vi "CALC_LIM_SEGM_AMPL_STOP.vi"(0 "VISA IN":refnum<visa-resource-name>, 1 "Segment number":i32, 2 "Stop number":i32, 5 "error in":errorcluster, 7 "Channel":i32) -> (14 "VISA Out":refnum<visa-resource-name>, 19 "error out":errorcluster)   [LabVIEW 2018, in "PNA-X.lvlib"]
doc: "CALCulate<cnum>:LIMit:SEGMent<snum>AMPLitude:STOP <num> \n(Read-Write) Sets the stop (end) of the Y-axis amplitude (response) value. \nSee Critical Note \nParameters \n<cnum> Channel number of the measurement. There must be a selected measurement \non that channel. If unspecified, <cnum> is set to 1. \n<snum> Segment number; if unspecified, value is set to 1. \n<num> Choose any number between: -500 and 500 \nDisplay value is limited to the Maximum and Minimum displayed Y-axis \nvalues. \nExamples CALC:LIM:SEGM1:AMPL:STOP 10 \ncalculate2:limit:segment2:amplitude:stop 10 \nQuery Syntax CALCulate<cnum>:LIMit:SEGMent<snum>AMPLitude:STOP? \nReturn Type Numeric \nDefault 0 \n1523"
uses:
  PNA-X.lvlib
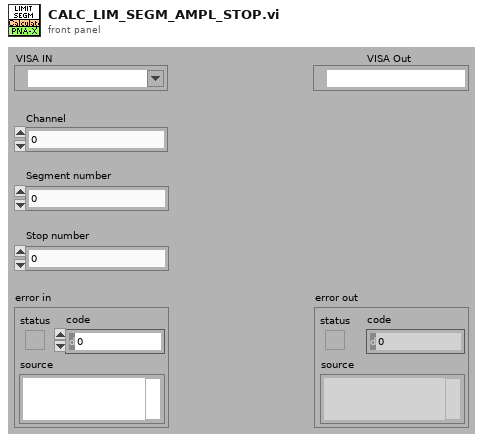
[diagram p1: front panel]
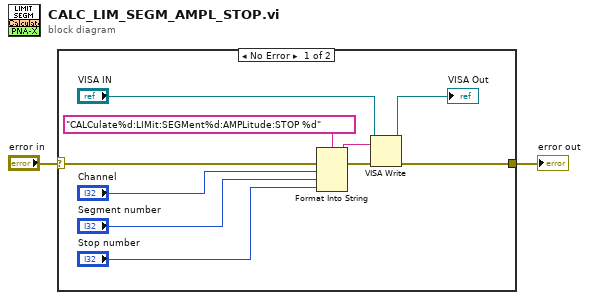
[diagram p0: block diagram]
diagram:
  n1 = case shown="No Error" "error in" {
    selector: "error in" -> [w12 w13]
    tunnel: [w7 w13] -> w1
    frame No Error {
      n2 = Format Into String(format string="CALCulate%d:LIMit:SEGMent%d:AMPLitude:STOP %d" ("Cmdline"), error in=w12, "Channel", "Segment number", "Stop number") -> (resulting string=w10:string, error out=w11:errorcluster)  [unwired: 1 in]
      n3 = VISA Write(VISA resource name="VISA IN", write buffer=w10, error in (no error)=w11) -> (VISA resource name out=→"VISA Out":refnum<visa-resource-name>, error out=w7:errorcluster)  [unwired: 1 out]
    }
    frame Error {
    }
  }
  "error out" <- w1
